vi "Stop Core.vi"(10 "final error code":i32, 11 "Nested in":refnum<class "UI Actor.lvclass">) -> (3 "Nested out":refnum<class "UI Actor.lvclass">)   [LabVIEW 2020, in "UI Actor.lvlib" / "UI Actor.lvclass"]
doc: "(<B>Filename</B>: Actor Framework.lvlib:Actor.lvclass:Stop Core.vi)\n\nDefines what the actor does before it stops. Use the <B>final error code</B> input to determine whether the actor shut down in response to an error.\n\nBy default, this method does nothing. A descendant class may override it to define behavior, such as shutting down any processes the actor initiated in its override of the Actor Core method."
uses:
  UI Actor.lvclass
  <vilib>/ActorFramework/Actor/Actor.lvclass
  UI Actor Messages/Close VISA Msg/Close VISA Msg.lvclass
  C:/Program Files/National Instruments/LabVIEW 2020/vi.lib/ActorFramework/Actor/Actor.lvclass
  C:/Users/Ceci Saldivar/Documents/ceci/7mo semestre/Henry/ya ultimo proyecto alv ptm/Proyecto-final-2000/UI Actor/UI Actor.lvclass
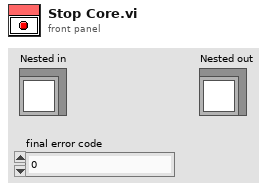
[diagram p1: front panel]
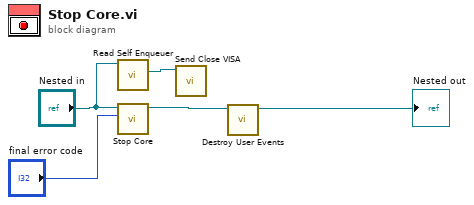
[diagram p0: block diagram]
diagram:
  n1 = call <vilib>:"Read Self Enqueuer.vi"("Actor"="Nested in") -> ("Self Enqueuer"=w1:refnum<class "Message Enqueuer.lvclass">)  [unwired: 10 in]
  n2 = call-parent "Stop Core.vi"("final error code"="final error code", "Actor in"="Nested in") -> ("Actor out"=w4:refnum<class "UI Actor.lvclass">)  [unwired: 9 in]
  n3 = call "Send Close VISA.vi"("Message Enqueuer"=w1) -> ()  [unwired: 9 in, 2 out]
  n4 = call "Destroy User Events.vi"("UI Template in"=w4) -> ("UI Template out"=→"Nested out":refnum<class "UI Actor.lvclass">)  [unwired: 10 in]
